vi "Sound Transmitter.vi"(8 "error in (no error)":errorcluster, 10 "String To Send":string) -> (0 "error out":errorcluster)   [LabVIEW 2025]
uses:
  LabVIEW/Globals/Cancelled Global.vi
  LabVIEW/Globals/Percent Complete Global.vi
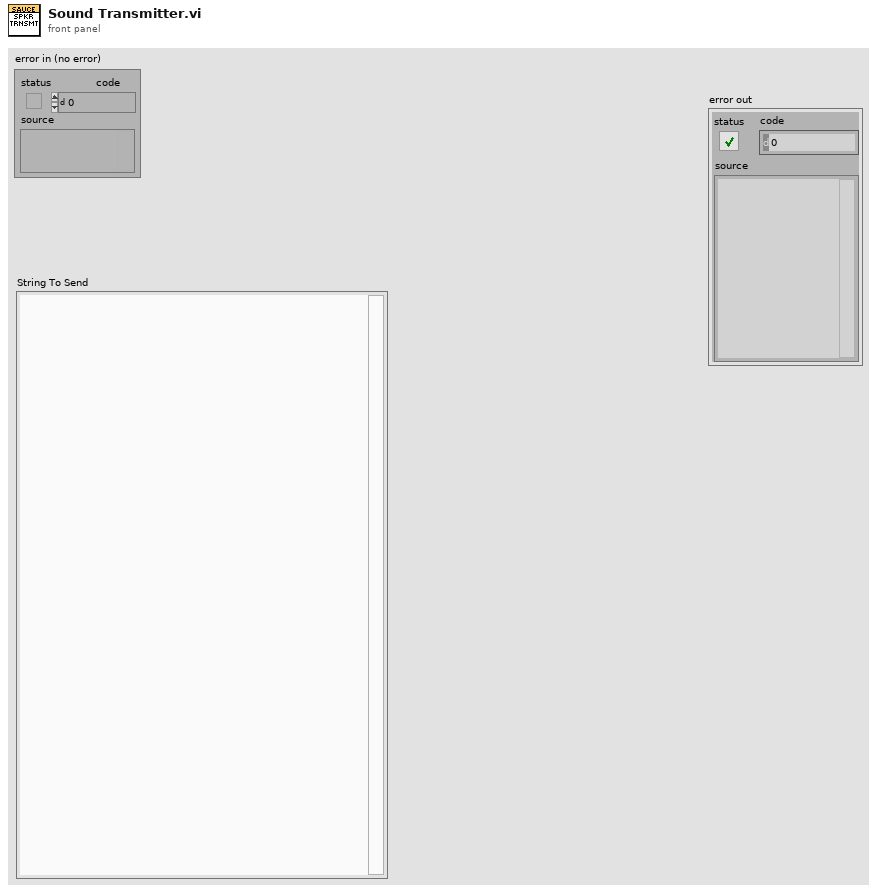
[diagram p1: front panel]
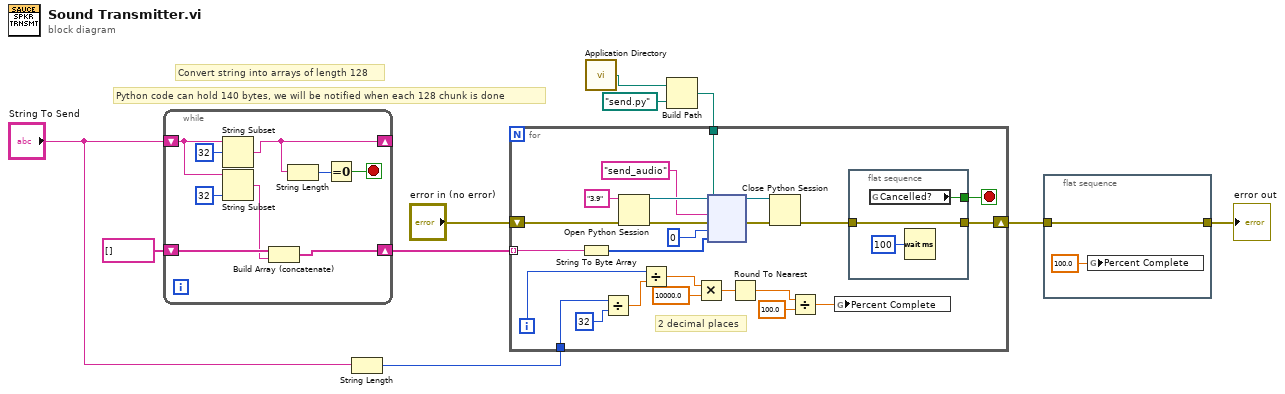
[diagram p0: block diagram]
diagram:
  # "Python code can hold 140 bytes, we will be notified when each 128 chunk is done"
  # "Convert string into arrays of length 128"
  n1 = while {
    shift-right: [w13] -> _
    shift-left: "String To Send" -> [w15]
    shift-right: [w16] -> w9
    shift-left: string[] [] ("Broken Up 64 Char Strings") -> [w17]
    stop <- w11 stop-if-true
    n2 = String Subset(string=w15, offset (0)=32) -> (substring=w13:string)  [unwired: 1 in]
    n3 = String Subset(string=w15, length (rest)=32 ("length (rest)")) -> (substring=w14:string)  [unwired: 1 in]
    n4 = Build Array (concatenate)(w17, w14) -> (w16:string[])
    n5 = String Length(string=w13) -> (length=w12:i32)
    n6 = Equal To 0?(x=w12) -> (x = 0?=w11:bool)
  }
  n7 = String Length(string="String To Send") -> (length=w7:i32)
  n8 = call <vilib>:"Application Directory.vi"() -> ("Application Directory"=w3:path)
  n9 = Build Path(base path=w3, name or relative path=path "send.py") -> (appended path=w1:path)
  n10 = for {
    tunnel: w9 -> [w25] mode=indexing
    shift-right: [w21] -> w4
    shift-left: "error in (no error)" -> [w26]
    tunnel: w7 -> [w41]
    tunnel: w1 -> [w27]
    i -> [w40]
    stop <- w22 stop-if-true
    # "2 decimal places"
    n11 = String To Byte Array(string=w25) -> (unsigned byte array=w24:u8[])
    n12 = Divide(x=w41, y=32) -> (x/y=w34:dbl)
    n13 = Open Python Session(python version="3.9" ("Python version"), 3:w26) -> (session out=w30:refnum<k35>, error out=w31:errorcluster)  [unwired: 1 in]
    n14 = Divide(x=w40, y=w34) -> (x/y=w39:dbl)
    n15 = Multiply(x=w39, y=10000.0) -> (x*y=w38:dbl)
    n16 = node(w30, w27, "send_audio" ("function name"), w31, 0, w24) -> (w33:refnum<k35>, w32:errorcluster)  [unwired: 2 in, 2 out]
    n17 = Round To Nearest(number=w38) -> (nearest integer value=w37:dbl)
    n18 = Close Python Session(session in=w33, error in=w32) -> (11:w20:errorcluster)
    n19 = Divide(x=w37, y=100.0) -> (x/y=w35:dbl)
    n20 = global write "Percent Complete Global.vi" "Percent Complete"(w35) -> ()
    n21 = flat-sequence {
      tunnel: [w46] -> w22
      tunnel: [w45] -> w21
      tunnel: w20 -> [w45]
      frame #0 {
        n22 = global read "Cancelled Global.vi" "Cancelled?"() -> (w46:bool)
        n23 = Wait (ms)(milliseconds to wait=u32 100) -> ()  [unwired: 1 out]
      }
    }
  }
  n24 = flat-sequence {
    tunnel: w4 -> [w47]
    tunnel: [w47] -> w6
    frame #0 {
      n25 = global write "Percent Complete Global.vi" "Percent Complete"(100.0 ("Percent Complete")) -> ()
    }
  }
  "error out" <- w6
